vi "Do.vi"(8 "error in (no error)":errorcluster, 10 "Actor in":refnum<class "Actor.lvclass">, 11 "Initialize UI Message":refnum<class "Initialize UI Message.lvclass">) -> (0 "error out":errorcluster, 2 "Actor out":refnum<class "Actor.lvclass">)   [LabVIEW 2017, in "Generic UI Actor.lvlib" / "Initialize UI Message.lvclass"]
uses:
  Initialize UI Message.lvclass
  <vilib>/ActorFramework/Actor/Actor.lvclass
  UI.lvclass
  C:/Program Files (x86)/National Instruments/LabVIEW 2017/vi.lib/ActorFramework/Actor/Actor.lvclass
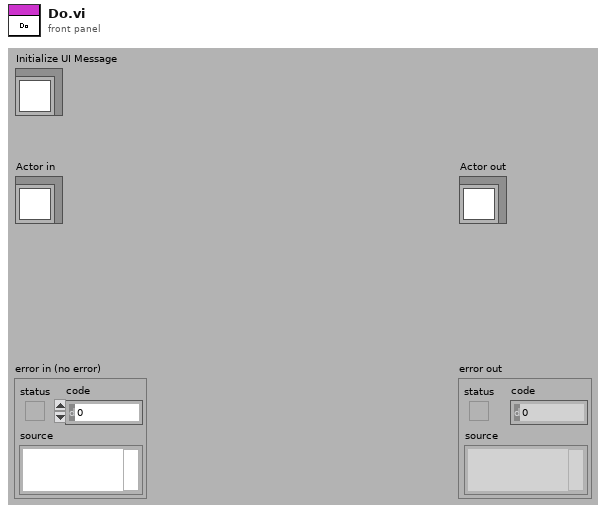
[diagram p1: front panel]
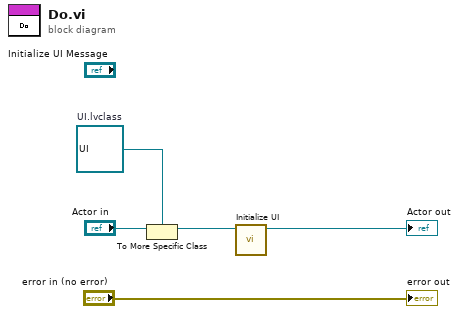
[diagram p0: block diagram]
diagram:
  w3 = refnum<class "UI.lvclass"> refnum  # UI.lvclass
  n1 = To More Specific Class(target class=w3, reference="Actor in") -> (specific class reference=w2:refnum<class "UI.lvclass">)  [unwired: 1 in, 1 out]
  n2 = call "Initialize UI.vi"("UI in"=w2) -> ("UI out"=→"Actor out":refnum<class "UI.lvclass">)  [unwired: 8 in, 2 out]
  "error out" <- "error in (no error)"
